vi "Merge Status.vi"(10 "New":T1=enum."Passed", 11 "Current":T1=enum."Passed") -> (1 "Changed?":bool, 3 "Merged":T1=enum."Passed")   [LabVIEW 2020, in "Method Result.lvlib"]
uses:
  Method Result.lvlib
  Core/Result/Status.ctl
  Core/Result/Result.lvlib
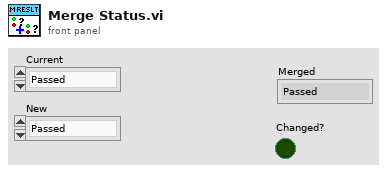
[diagram p1: front panel]
types:
  T1 = typedef "Result.lvlib/Status.ctl" = enum16{"", "Passed", "Failed", "Error", "Skipped", "Setup Error", "Broken", "Teardown Error"}
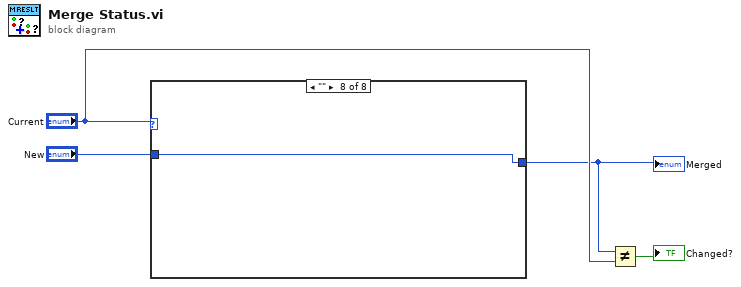
[diagram p0: block diagram]
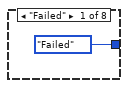
[diagram p3: hidden frame]
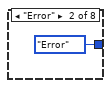
[diagram p4: hidden frame]
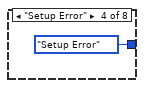
[diagram p5: hidden frame]
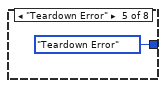
[diagram p6: hidden frame]
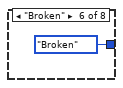
[diagram p7: hidden frame]
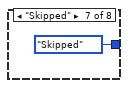
[diagram p8: hidden frame]
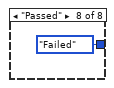
[diagram p9: hidden frame]
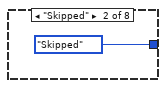
[diagram p10: hidden frame]
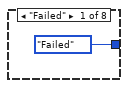
[diagram p12: hidden frame]
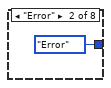
[diagram p13: hidden frame]
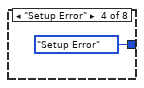
[diagram p14: hidden frame]
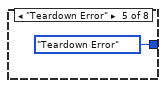
[diagram p15: hidden frame]
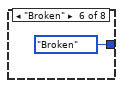
[diagram p16: hidden frame]
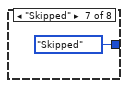
[diagram p17: hidden frame]
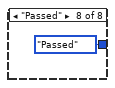
[diagram p18: hidden frame]
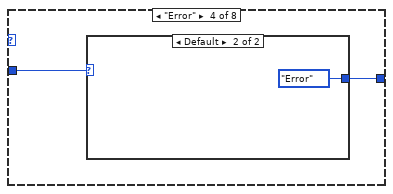
[diagram p19: hidden frame]
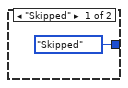
[diagram p20: hidden frame]
diagram:
  n1 = case shown="\"\"" "Current" {
    selector: "Current" -> [w5 _ w17 _ _ _ _ _]
    tunnel: "New" -> [w7 _ w19 w28 w32 w36 w40 w44]
    tunnel: [w6 Status."Skipped" ("Merged Status") w18 w29 w33 w37 w41 w44] -> w2
    frame "Failed" {
      n2 = case shown="\"\"" w7 {
        tunnel: [Status."Failed" ("Merged Status") Status."Error" ("Merged Status") w10 Status."Setup Error" ("Merged Status") Status."Teardown Error" ("Merged Status") Status."Broken" ("Merged Status") Status."Skipped" ("Merged Status") Status."Failed" ("Merged Status")] -> w6
        tunnel: w5 -> [_ _ w10 _ _ _ _ _]
        frame "Failed" {
        }
        frame "Error" {
        }
        frame "" {
        }
        frame "Setup Error" {
        }
        frame "Teardown Error" {
        }
        frame "Broken" {
        }
        frame "Skipped" {
        }
        frame "Passed" {
        }
      }
    }
    frame "Skipped" {
    }
    frame "Passed" {
      n3 = case shown="\"\"" w19 {
        tunnel: [Status."Failed" ("Merged Status") Status."Error" ("Merged Status") w22 Status."Setup Error" ("Merged Status") Status."Teardown Error" ("Merged Status") Status."Broken" ("Merged Status") Status."Skipped" ("Merged Status") Status."Passed" ("Merged Status")] -> w18
        tunnel: w17 -> [_ _ w22 _ _ _ _ _]
        frame "Failed" {
        }
        frame "Error" {
        }
        frame "" {
        }
        frame "Setup Error" {
        }
        frame "Teardown Error" {
        }
        frame "Broken" {
        }
        frame "Skipped" {
        }
        frame "Passed" {
        }
      }
    }
    frame "Error" {
      n4 = case shown="Default" w28 {
        tunnel: [Status."Skipped" ("Merged Status") Status."Error" ("Merged Status")] -> w29
        frame "Skipped" {
        }
        frame Default {
        }
      }
    }
    frame "Setup Error" {
      n5 = case shown="Default" w32 {
        tunnel: [Status."Skipped" ("Merged Status") Status."Setup Error" ("Merged Status")] -> w33
        frame "Skipped" {
        }
        frame Default {
        }
      }
    }
    frame "Broken" {
      n6 = case shown="Default" w36 {
        tunnel: [Status."Broken" ("Merged Status") Status."Setup Error" ("Merged Status")] -> w37
        frame Default {
        }
        frame "Setup Error" {
        }
      }
    }
    frame "Teardown Error" {
      n7 = case shown="Default" w40 {
        tunnel: [Status."Skipped" ("Merged Status") Status."Teardown Error" ("Merged Status")] -> w41
        frame "Skipped" {
        }
        frame Default {
        }
      }
    }
    frame "" {
    }
  }
  "Merged" <- w2
  n8 = Not Equal?(x=w2, y="Current") -> (x != y?=→"Changed?":bool)
